vi "PT2.vi"(0 "input u(k)":dbl, 5 "G":dbl, 7 "T1":dbl, 9 "T2":dbl, 11 "error in (no error)":errorcluster) -> (6 "output y(k)":dbl, 15 "error out":errorcluster)   [LabVIEW 2022 SP3]
uses:
  <vilib>/addons/Control Design/_Model Construction/Model Typedefs.llb/CD Transfer Function Model (SISO).ctl
  <vilib>/addons/System Identification/Model Typedefs.llb/si_Bode Magnitude Plot.ctl
  <vilib>/addons/System Identification/Model Typedefs.llb/si_Bode Phase Plot.ctl
  <vilib>/Simulation/DiscreteLinear/Implementation/NILVSim Discrete Transfer Function Direct.llb/SIM Discrete Transfer Function Diagram (SISO CD).vi
  <vilib>/Simulation/ContinuousLinear/Implementation/Shared/SIM Transfer Function Support.llb/SIM Convert CD TF to SIM (SISO).vi
  <vilib>/Simulation/ContinuousLinear/Implementation/Shared/SIM Transfer Function Support.llb/SIM TransferFunction Normalize to Buffer.vi
  <vilib>/Simulation/DiscreteLinear/Implementation/Shared/SIM Init Discrete States.vi
  <vilib>/Simulation/DiscreteLinear/Implementation/NILVSim Discrete Transfer Function Direct.llb/SIM Transfer Function Direct core (SISO).vi
  <vilib>/Simulation/ContinuousLinear/Implementation/Shared/SIM Transfer Function Support.llb/SIM TransferFunction Normalize.vi
  <vilib>/Simulation/Implementation/Shared/SIM Polynomials.llb/SIM Remove Zero Coefficients (DBL).vi
  <vilib>/addons/Control Design/_Frequency Response Analysis/Frequency Response.llb/Frequency Response subVI/cd_Bode (Transfer Function).vi
  <vilib>/Simulation/Implementation/Shared/SIM Polynomials.llb/SIM Divide Polynomials (DBL).vi
  <vilib>/Simulation/Implementation/Shared/SIM BuildSimErr.vi
  <vilib>/Simulation/Implementation/XNodeFramework/SimXNode/SimX.xnode
  <vilib>/addons/Control Design/_Model Construction/Model Typedefs.llb/CD Transfer Function Model (MIMO).ctl
  <vilib>/addons/Control Design/_Model Construction/Model Typedefs.llb/CD General Elements.ctl
  <vilib>/addons/Control Design/_Model Construction/NI_LinSys_Model Typedefs.lvlib
  <vilib>/addons/Control Design/_Frequency Response Analysis/NI_CD_Frequency Response.lvlib
  <vilib>/addons/System Identification/NI_SysID.lvlib
panel:
  out "Bode Phase Plot":T1
  out "Bode Magnitude Plot":T2
  out "Step Response Graph":cluster{"time":dbl[], dbl[]}[](graph)
  out "S Transf":picture
  in  "initialize":bool
  out "element":T3 {"delay" format="%.4f"; "Denominator" format="%#_3g"; "Numerator" format="%#_3g"}
  out "Z Transf":picture
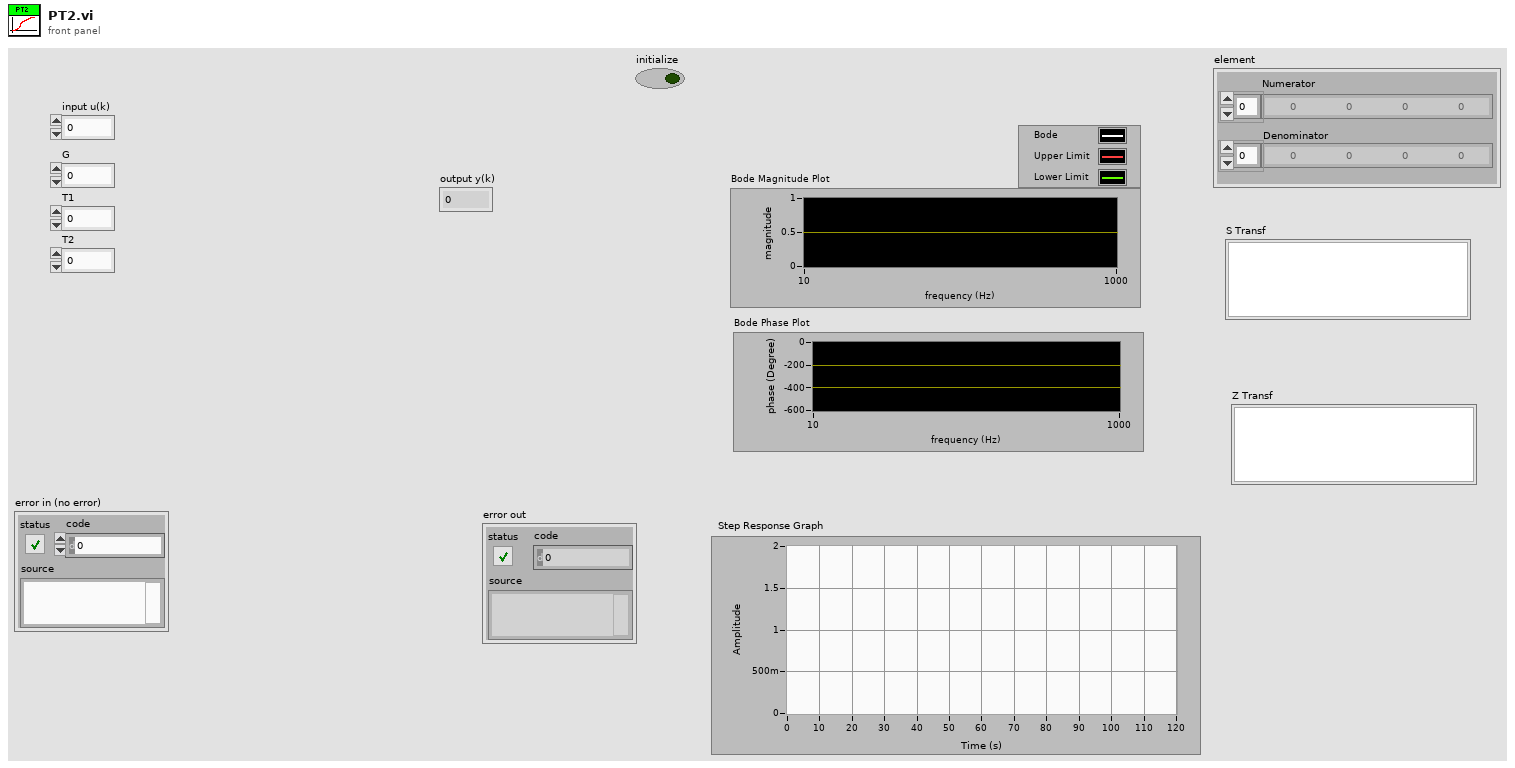
[diagram p1: front panel]
types:
  T1 = typedef "NI_SysID.lvlib/si_Bode Phase Plot.ctl" = cluster{"frequency":dbl[], "amplitude":dbl[]}[]
  T2 = typedef "NI_SysID.lvlib/si_Bode Magnitude Plot.ctl" = cluster{"frequency":dbl[], "amplitude":dbl[]}[]
  T3 = typedef "NI_LinSys_Model Typedefs.lvlib/CD Transfer Function Model (SISO).ctl" = cluster{"Numerator":dbl[], "Denominator":dbl[], "delay":dbl}
  T4 = typedef "NI_LinSys_Model Typedefs.lvlib/CD Transfer Function Model (MIMO).ctl" = cluster{"properties":T5, "transfer function(s)":T3[][]}
  T5 = typedef "NI_LinSys_Model Typedefs.lvlib/CD General Elements.ctl" = cluster{"Model name":string, "Input names":string[], "Output names":string[], "Input Delays":dbl[], "Output Delays":dbl[], "Sampling Time":dbl, "Notes":string}
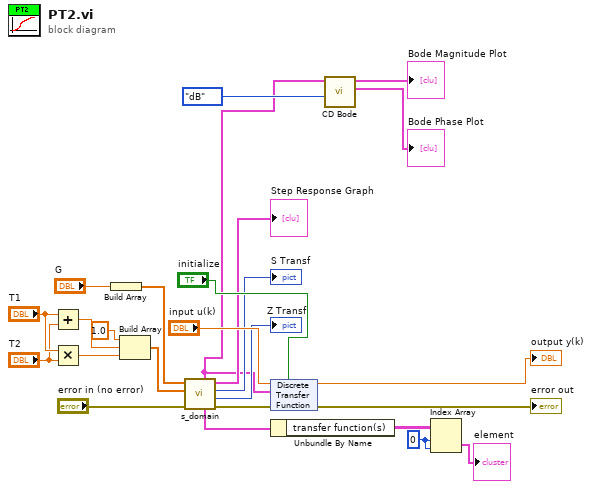
[diagram p0: block diagram]
diagram:
  w7 = 0 ("index (row)")
  n1 = Add(x="T1", y="T2") -> (x+y=w18:dbl)
  n2 = Multiply(x="T1", y="T2") -> (x*y=w15:dbl)
  n3 = Build Array("G") -> (w14:dbl[])
  n4 = Build Array(1.0 ("element"), w18, w15) -> (w13:dbl[])
  n5 = call "s_domain.vi"("error in (no error)"="error in (no error)", "Denominator"=w13, "Numerator"=w14) -> ("error out"=w3:errorcluster, "z-domain"=→"Z Transf":picture, "s-domain"=→"S Transf":picture, "Step Response Graph"=→"Step Response Graph":cluster{"time":dbl[], dbl[]}[], "Discrete Transfer Function Model"=w6:T4, "Transfer Function Model"=w4:T4)  [unwired: 3 in]
  n6 = xnode "Discrete Transfer Function"("input u(k)"="input u(k)", "Transfer Function"=w4, "initialize"="initialize", "error in (no error)"=w3) -> ("output y(k)"=→"output y(k)":dbl, "error out"=→"error out":errorcluster)
  n7 = Unbundle By Name(w6) -> ("transfer function(s)"=w8:T3[][])
  n8 = call-poly <vilib>:"CD Bode.vi"("Magnitude Scale"=enum16{"linear", "dB"}."dB", "Transfer Function Model"=w4) -> ("Bode Phase"=→"Bode Phase Plot":cluster{"W":dbl[], "Magnitude":dbl[]}[], "Bode Magnitude"=→"Bode Magnitude Plot":cluster{"W":dbl[], "Magnitude":dbl[]}[])  [unwired: 5 in, 3 out]
  n9 = Index Array(array=w8, index (row)=w7, index (col)=w7) -> (element=→"element":T3)
